vi "Read Time Instant.vi"(8 "error in (no error)":errorcluster, 10 "Reference Level (0)":dbl, 11 "VISA resource name":refnum<visa-resource-name>) -> (0 "error out":errorcluster, 1 "Time Instant Data":dbl[](array[numeric]), 2 "Time Instant":dbl, 3 "VISA resource name out":refnum<visa-resource-name>)   [LabVIEW 2014, in "Agilent U2000 Series.lvlib"]
doc: "Returns the time instant array at which the power waveform intersects the reference level supplied as the command parameter. This allows the time instant used to calculate the pulse parameters to be found. It also allows the calculation of the transition between non- standard reference levels.\n\nNote:\nIn case of U2040 X-Series, it is applicable for U2042XA/U2044XA/U2049XA only."
uses:
  Agilent U2000 Series.lvlib
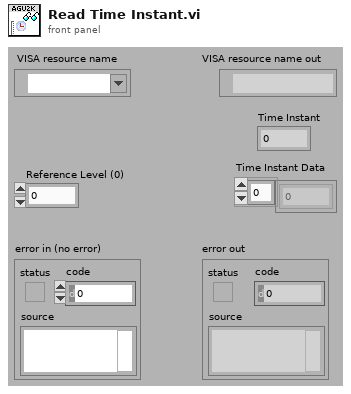
[diagram p1: front panel]
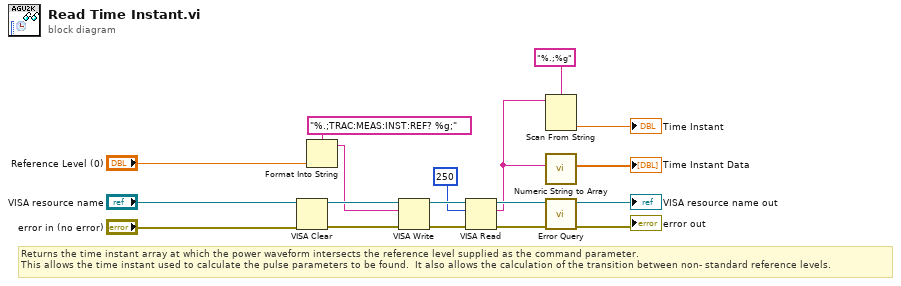
[diagram p0: block diagram]
diagram:
  # "Returns the time instant array at which the power waveform intersects the reference level supplied as the command parameter. \nThis allows the time instant used to calculate the pulse parameters to be found.  It also allows the calculation of the transition between non- standard reference levels."
  n1 = VISA Clear(VISA resource name="VISA resource name", error in (no error)="error in (no error)") -> (VISA resource name out=w16:refnum<visa-resource-name>, error out=w15:errorcluster)
  n2 = Format Into String(format string="%.;TRAC:MEAS:INST:REF? %g;", "Reference Level (0)") -> (resulting string=w11:string)  [unwired: 2 in, 1 out]
  n3 = VISA Write(VISA resource name=w16, write buffer=w11, error in (no error)=w15) -> (VISA resource name out=w14:refnum<visa-resource-name>, error out=w13:errorcluster)  [unwired: 1 out]
  n4 = VISA Read(VISA resource name=w14, byte count=u32 250, error in (no error)=w13) -> (VISA resource name out=w5:refnum<visa-resource-name>, read buffer=w1:string, error out=w6:errorcluster)  [unwired: 1 out]
  n5 = Scan From String(format string="%.;%g", input string=w1) -> (output 1=→"Time Instant":dbl)  [unwired: 2 in, 4 out]
  n6 = call "Numeric String to Array.vi"("Sheet String"=w1) -> ("Table Array"=→"Time Instant Data":dbl[])  [unwired: 8 in]
  n7 = call "Error Query.vi"("error in (no error)"=w6, "VISA resource name"=w5) -> ("error out"=→"error out":errorcluster, "VISA resource name out"=→"VISA resource name out":refnum<visa-resource-name>)  [unwired: 8 out]
